vi "solar_type Get Items (Ctrl).vi"(4 "Include Cluster Prefix? (F)":bool, 6 "Prefix":string, 8 "error in (no error)":errorcluster, 11 "Ctl Refnum":refnum<vi>) -> (0 "error out":errorcluster, 1 "Ctrl Name":string, 2 "Ctrl Type":T1, 3 "Items":T2[](array[typedef]), 5 "Ctrl Variant":variant)   [LabVIEW 2018]
doc: "This gets the control parameters as a variant array."
uses:
  solar_type Item Type.ctl
  solar_type Item.ctl
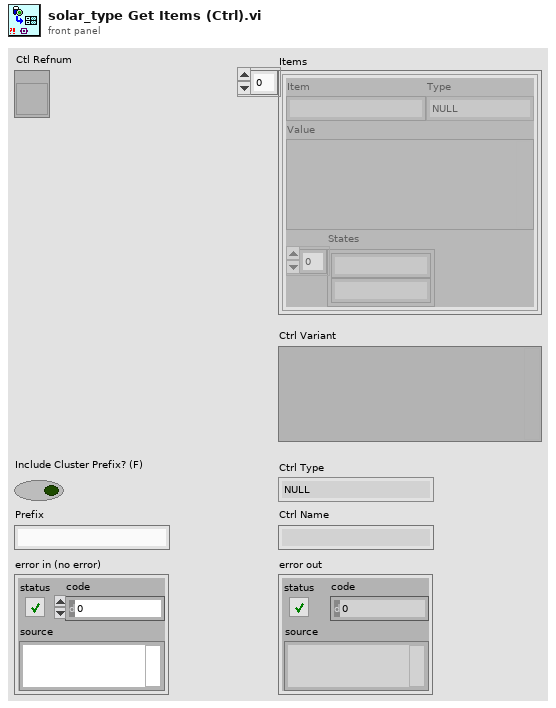
[diagram p1: front panel]
types:
  T1 = typedef "solar_type Item Type.ctl" = enum16{"NULL", "UNKNOWN", "CLUSTER", "I8", "I16", "I32", "I64", "U8", "U16", "U32", "U64", "U8_ENUM", "U16_ENUM", "U32_ENUM", "SGL", "DBL", "BOOLEAN", "STRING", "PATH", "VISA", "TAG", "TIME", "I8_1D", "I16_1D", "I32_1D", "I64_1D", "U8_1D", "U16_1D", "U32_1D", "U64_1D", "U8_ENUM_1D", "U16_ENUM_1D", "U32_ENUM_1D", "SGL_1D", "DBL_1D", "BOOLEAN_1D", "STRING_1D", "PATH_1D", "VISA_1D", "TAG_1D", "TIME_1D", "I8_2D", "I16_2D", "I32_2D", "I64_2D", "U8_2D", "U16_2D", "U32_2D", "U64_2D", "U8_ENUM_2D", "U16_ENUM_2D", "U32_ENUM_2D", "SGL_2D", "DBL_2D", "BOOLEAN_2D", "STRING_2D", "PATH_2D", "VISA_2D", "TAG_2D", "TIME_2D"}
  T2 = typedef "solar_type Item.ctl" = cluster{"Item":string, "Type":T1, "Value":variant, "States":string[]}
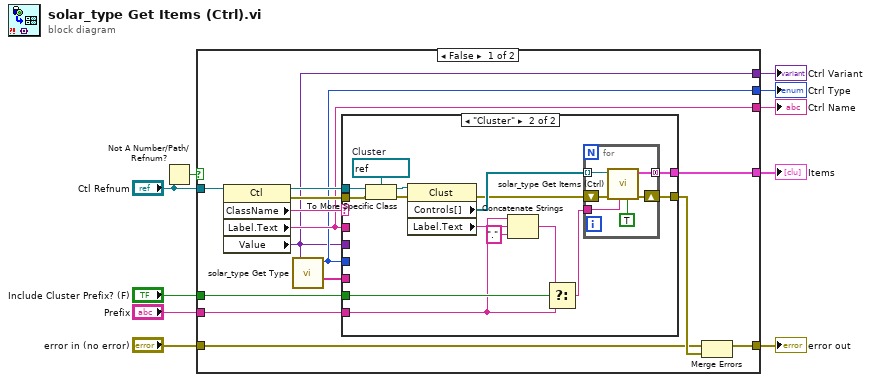
[diagram p0: block diagram]
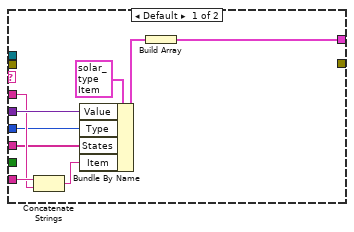
[diagram p2: hidden frame]
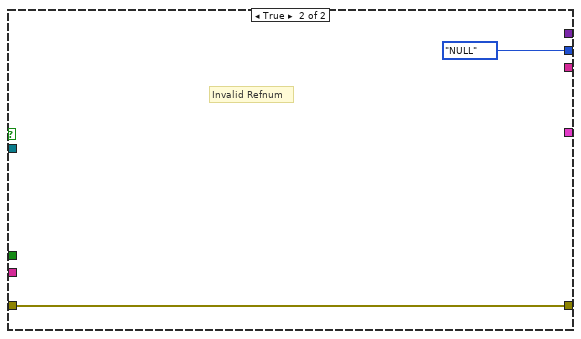
[diagram p3: hidden frame]
diagram:
  n1 = Not A Number/Path/Refnum?(number/path/refnum="Ctl Refnum") -> (NaN/Path/Refnum?=w3:bool)
  n2 = case shown="False" w3 {
    tunnel: "Include Cluster Prefix? (F)" -> [w24 _]
    tunnel: "Prefix" -> [w23 _]
    tunnel: "Ctl Refnum" -> [w22 _]
    tunnel: [w21 _] -> w8
    tunnel: [w17 _] -> w7
    tunnel: [w16 solar_type_Item_Type."NULL" ("Type")] -> w6
    tunnel: [w14 _] -> w5
    tunnel: "error in (no error)" -> [w12 w55]
    tunnel: [w11 w55] -> w1
    frame False {
      n3 = property class="Ctl"(reference=w22) -> (reference out=w20:refnum<vi>, error out=w18:errorcluster, "ClassName"=w19:string, "Label.Text"=w17:string, "Value"=w14:variant)  [unwired: 1 in]
      n4 = call "solar_type Get Type.vi"("Variant"=w14) -> ("Type"=w16:T1, "Enum Names"=w15:string[])  [unwired: 4 in, 1 out]
      n5 = case shown="\"Cluster\"" w19 {
        tunnel: w20 -> [_ w41]
        tunnel: w24 -> [_ w48]
        tunnel: w23 -> [w33 w44]
        tunnel: [w30 w43] -> w21
        tunnel: [_ w42] -> w13
        tunnel: w18 -> [_ w37]
        tunnel: w14 -> [w28 _]
        tunnel: w17 -> [w27 _]
        tunnel: w16 -> [w26 _]
        tunnel: w15 -> [w25 _]
        frame Default {
          n6 = Concatenate Strings(w33, w27) -> (w29:string)
          n7 = Bundle By Name(cluster=T2 {"Item"="", "Type"=enum."NULL", "Value"=variant, "States"=[]} ("Item"), "Value"=w28, "Type"=w26, "States"=w25, "Item"=w29) -> (w31:T2)
          n8 = Build Array(w31) -> (w30:T2[])
        }
        frame "Cluster" {
          w38 = refnum<vi> refnum  # Cluster
          n9 = To More Specific Class(target class=w38, reference=w41, error in=w37) -> (specific class reference=w39:refnum<vi>, error out=w36:errorcluster)
          n10 = property class="Clust"(reference=w39, error in=w36) -> (error out=w34:errorcluster, "Controls[]"=w35:refnum<vi>[], "Label.Text"=w40:string)  [unwired: 1 out]
          n11 = Concatenate Strings(w44, w40, "." ("string")) -> (w46:string)
          n12 = Select(t=w46, s=w48, f=w44) -> (s? t:f=w45:string)
          n13 = for {
            tunnel: w35 -> [w54] mode=indexing
            tunnel: w45 -> [w50]
            tunnel: [w51] -> w43 mode=concatenating
            shift-right: [w52] -> w42
            shift-left: w34 -> [w53]
            n14 = call "solar_type Get Items (Ctrl).vi"("Include Cluster Prefix? (F)"=TRUE, "Prefix"=w50, "error in (no error)"=w53, "Ctl Refnum"=w54) -> ("error out"=w52:errorcluster, "Items"=w51:T2[])  [unwired: 3 in, 3 out]
          }
        }
      }
      n15 = Merge Errors(w12, w13) -> (w11:errorcluster)
    }
    frame True {
      # "Invalid Refnum"
    }
  }
  "Items" <- w8
  "error out" <- w1
  "Ctrl Name" <- w7
  "Ctrl Type" <- w6
  "Ctrl Variant" <- w5
